vi "Арифметика5.vi"(3 "B":T3, 4 "Func":T2, 5 "A":T4) -> (0 "Result":T1, 1 "C":bool, 2 "Type":bool)   [LabVIEW 2017]
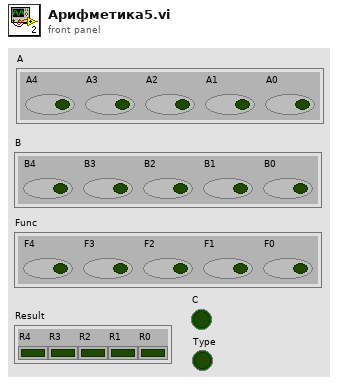
[diagram p1: front panel]
types:
  T1 = cluster{"R4":bool, "R3":bool, "R2":bool, "R1":bool, "R0":bool}
  T2 = cluster{"F4":bool, "F3":bool, "F2":bool, "F1":bool, "F0":bool}
  T3 = cluster{"B4":bool, "B3":bool, "B2":bool, "B1":bool, "B0":bool}
  T4 = cluster{"A4":bool, "A3":bool, "A2":bool, "A1":bool, "A0":bool}
  T5 = cluster{"SUM":bool, "SUM":bool, "SUM":bool, "SUM":bool, "SUM":bool}
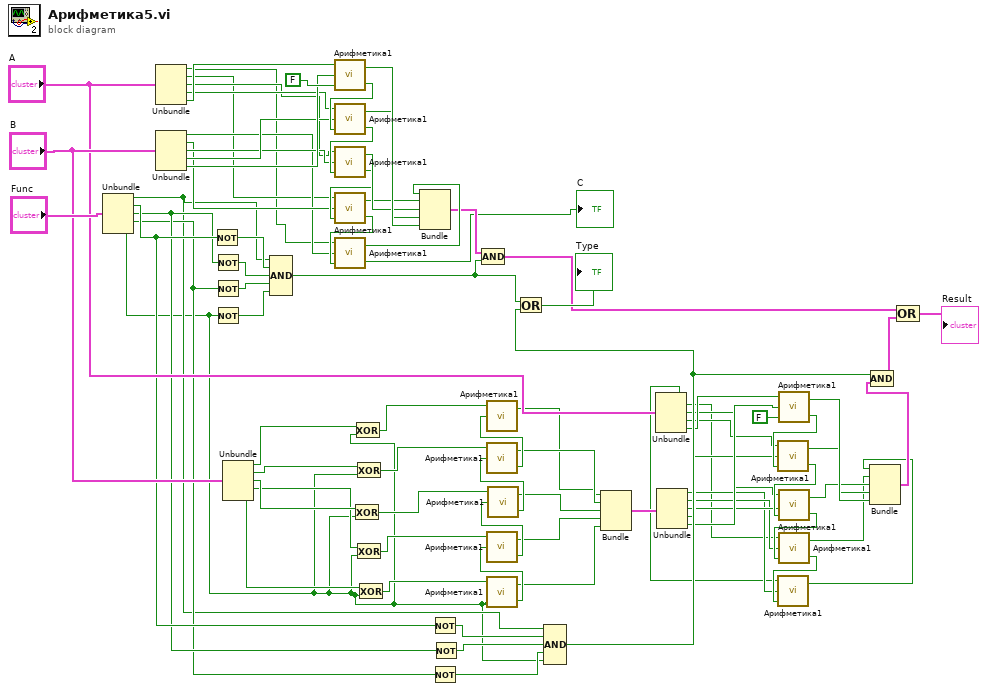
[diagram p0: block diagram]
diagram:
  n1 = Unbundle("Func") -> ("F4"=w28:bool, "F3"=w31:bool, "F2"=w30:bool, "F1"=w29:bool, "F0"=w24:bool)
  n2 = Unbundle("A") -> ("A4"=w60:bool, "A3"=w61:bool, "A2"=w62:bool, "A1"=w63:bool, "A0"=w79:bool)
  n3 = Unbundle("B") -> ("B4"=w64:bool, "B3"=w65:bool, "B2"=w66:bool, "B1"=w75:bool, "B0"=w77:bool)
  n4 = Not(x=w31) -> (.not. x?=w83:bool)
  n5 = Not(x=w30) -> (.not. x?=w82:bool)
  n6 = Not(x=w29) -> (.not. x?=w81:bool)
  n7 = Not(x=w24) -> (.not. x?=w80:bool)
  n8 = Unbundle("B") -> ("B4"=w52:bool, "B3"=w51:bool, "B2"=w50:bool, "B1"=w48:bool, "B0"=w49:bool)
  n9 = Compound Arithmetic op=AND(w28, w83, w82, w81, w80) -> (w57:bool)
  n10 = call "Арифметика1.vi"("C"=FALSE, "B"=w77, "A"=w79) -> ("C"=w76:bool, "SUM"=w74:bool)
  n11 = call "Арифметика1.vi"("C"=w76, "B"=w75, "A"=w63) -> ("C"=w69:bool, "SUM"=w73:bool)
  n12 = call "Арифметика1.vi"("C"=w69, "B"=w66, "A"=w62) -> ("C"=w68:bool, "SUM"=w72:bool)
  n13 = call "Арифметика1.vi"("C"=w68, "B"=w65, "A"=w61) -> ("C"=w67:bool, "SUM"=w71:bool)
  n14 = call "Арифметика1.vi"("C"=w67, "B"=w64, "A"=w60) -> ("C"=→"C":bool, "SUM"=w70:bool)
  n15 = Exclusive Or(1:w24, 2:w50) -> (0:w40:bool)
  n16 = Exclusive Or(1:w24, 2:w52) -> (0:w38:bool)
  n17 = Exclusive Or(1:w24, 2:w51) -> (0:w39:bool)
  n18 = Exclusive Or(1:w24, 2:w48) -> (0:w41:bool)
  n19 = Exclusive Or(1:w24, 2:w49) -> (0:w42:bool)
  n20 = Bundle("SUM"=w70, "SUM"=w71, "SUM"=w72, "SUM"=w73, "SUM"=w74) -> (w59:T5)  [unwired: 1 in]
  n21 = Not(x=w31) -> (.not. x?=w27:bool)
  n22 = Not(x=w29) -> (.not. x?=w25:bool)
  n23 = Not(x=w30) -> (.not. x?=w26:bool)
  n24 = Compound Arithmetic op=AND(w59, w57) -> (w54:T5)
  n25 = call "Арифметика1.vi"("C"=w24, "A"=w42) -> ("C"=w44:bool, "SUM"=w37:bool)  [unwired: 1 in]
  n26 = call "Арифметика1.vi"("B"=w44, "A"=w41) -> ("C"=w45:bool, "SUM"=w36:bool)  [unwired: 1 in]
  n27 = call "Арифметика1.vi"("B"=w45, "A"=w40) -> ("C"=w46:bool, "SUM"=w35:bool)  [unwired: 1 in]
  n28 = call "Арифметика1.vi"("B"=w46, "A"=w39) -> ("C"=w47:bool, "SUM"=w34:bool)  [unwired: 1 in]
  n29 = call "Арифметика1.vi"("B"=w47, "A"=w38) -> ("SUM"=w33:bool)  [unwired: 1 in, 1 out]
  n30 = Compound Arithmetic op=AND(w28, w27, w26, w25, w24) -> (w23:bool)
  n31 = Or(x=w57, y=w23) -> (x .or. y?=→"Type":bool)
  n32 = Bundle("SUM"=w33, "SUM"=w34, "SUM"=w35, "SUM"=w36, "SUM"=w37) -> (w32:T5)  [unwired: 1 in]
  n33 = Unbundle("A") -> ("A4"=w6:bool, "A3"=w7:bool, "A2"=w8:bool, "A1"=w9:bool, "A0"=w18:bool)
  n34 = Unbundle(w32) -> ("SUM"=w10:bool, "SUM"=w11:bool, "SUM"=w12:bool, "SUM"=w13:bool, "SUM"=w19:bool)
  n35 = call "Арифметика1.vi"("C"=FALSE, "B"=w19, "A"=w18) -> ("C"=w17:bool, "SUM"=w5:bool)
  n36 = call "Арифметика1.vi"("C"=w17, "B"=w13, "A"=w9) -> ("C"=w16:bool, "SUM"=w4:bool)
  n37 = call "Арифметика1.vi"("C"=w16, "B"=w12, "A"=w8) -> ("C"=w15:bool, "SUM"=w3:bool)
  n38 = call "Арифметика1.vi"("C"=w15, "B"=w11, "A"=w7) -> ("C"=w14:bool, "SUM"=w2:bool)
  n39 = call "Арифметика1.vi"("C"=w14, "B"=w10, "A"=w6) -> ("SUM"=w1:bool)  [unwired: 1 out]
  n40 = Bundle("SUM"=w1, "SUM"=w2, "SUM"=w3, "SUM"=w4, "SUM"=w5) -> (w22:T5)  [unwired: 1 in]
  n41 = Compound Arithmetic op=AND(w23, w22) -> (w21:T5)
  n42 = Compound Arithmetic op=OR(w54, w21) -> (→"Result":T5)
